vi "Test Compare Unequal Timestamps.vi"(8 "error in (no error)":errorcluster, 11 "Comparison Test Double in":refnum<class "Comparison Test Double.lvclass">) -> (0 "error out":errorcluster, 3 "Comparison Test Double out":refnum<class "Comparison Test Double.lvclass">)   [LabVIEW 2020, in "Comparison Test Double.lvclass"]
uses:
  Comparison Test Double.lvclass
  D:/git/astemes-lunit/source/LUnit Test Case.lvclass
  source/LUnit Test Case.lvclass/LUnit Test Case.ctl
  Comparison Test Double.lvclass/Comparison Test Double.ctl
  23615402-9b1f-4bd5-97a8-ca362d09ae43.vi
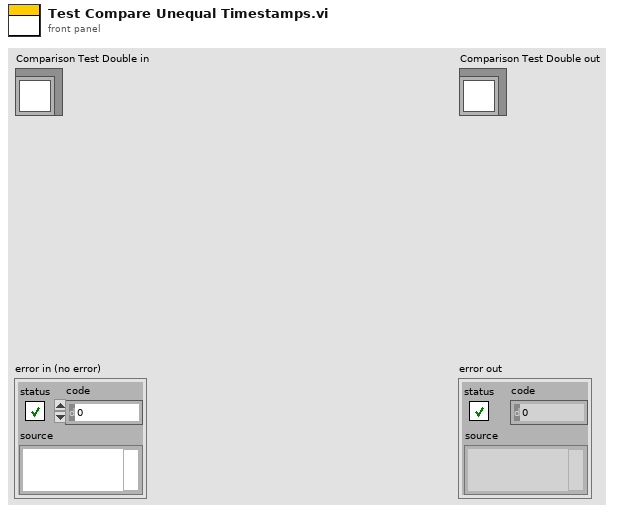
[diagram p1: front panel]
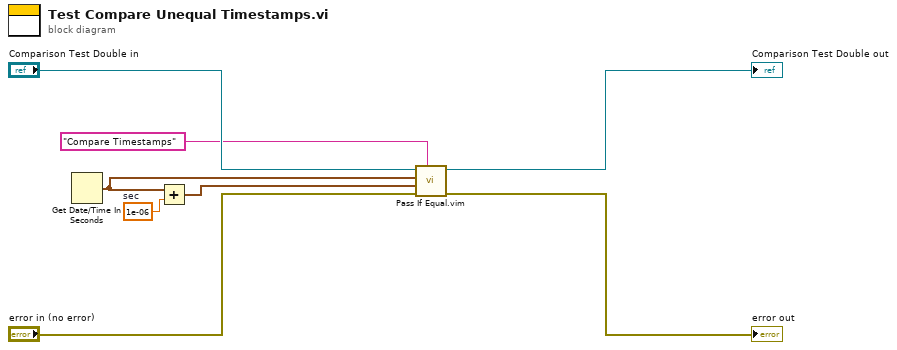
[diagram p0: block diagram]
diagram:
  w1 = 1e-06  # sec
  n1 = Get Date/Time In Seconds() -> (seconds since 1Jan1904=w3:timestamp)
  n2 = Add(x=w3, y=w1) -> (x+y=w2:timestamp)
  n3 = call "Pass If Equal.vim"("Description"="Compare Timestamps", "error in (no error)"="error in (no error)", "Actual"=w2, "Expected"=w3, "LUnit Test Case In"="Comparison Test Double in") -> ("error out"=→"error out":errorcluster, "LUnit Test Case Out"=→"Comparison Test Double out":refnum<class "Comparison Test Double.lvclass">)  [unwired: 5 in]
